vi "Access Privilege_Enable Disable Control.vi"(10 "Sidebar Ref":refnum<vi>, 11 "Previllage":string) -> ()   [LabVIEW 2023, in "GUI.lvlib"]
uses:
  GUI.lvlib
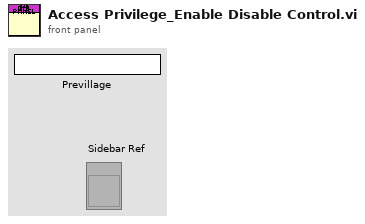
[diagram p1: front panel]
types:
  T1 = enum8{"Enabled", "Disabled", "Disabled and Grayed Out"}
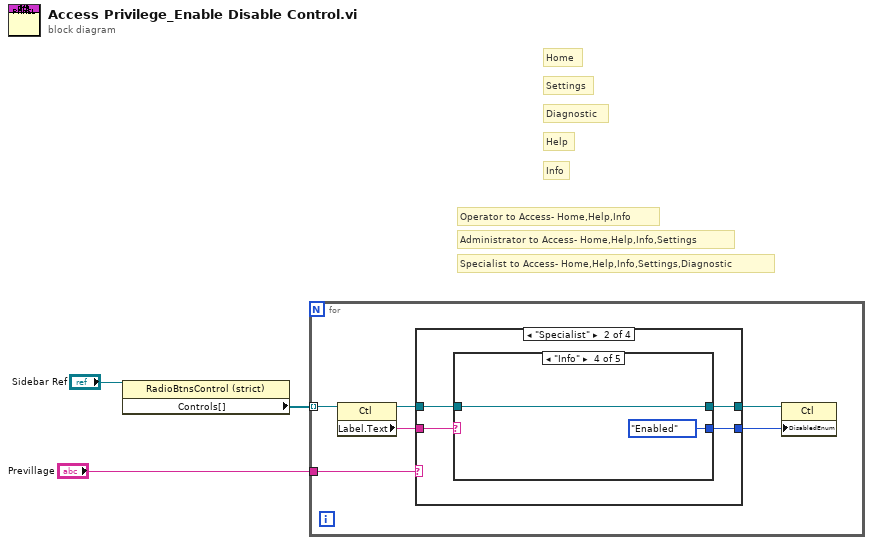
[diagram p0: block diagram]
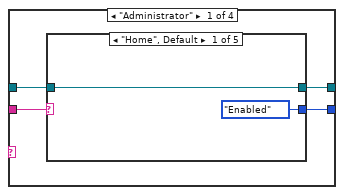
[diagram p2: hidden frame]
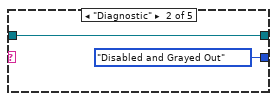
[diagram p3: hidden frame]
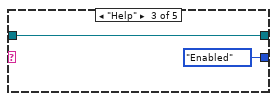
[diagram p4: hidden frame]
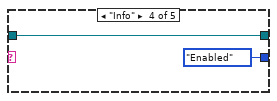
[diagram p5: hidden frame]
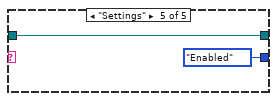
[diagram p6: hidden frame]
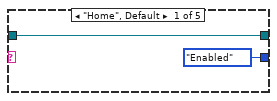
[diagram p7: hidden frame]
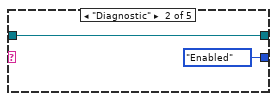
[diagram p8: hidden frame]
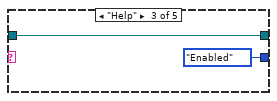
[diagram p9: hidden frame]
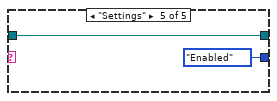
[diagram p10: hidden frame]
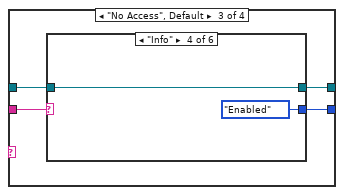
[diagram p11: hidden frame]
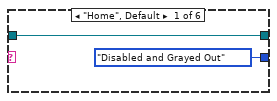
[diagram p12: hidden frame]
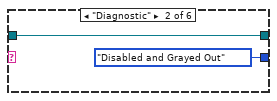
[diagram p13: hidden frame]
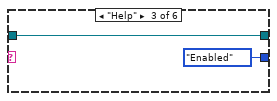
[diagram p14: hidden frame]
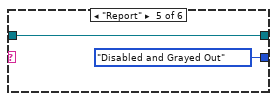
[diagram p15: hidden frame]
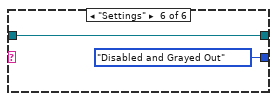
[diagram p16: hidden frame]
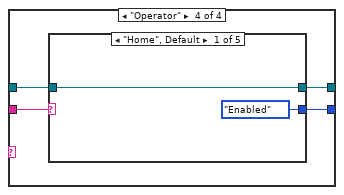
[diagram p17: hidden frame]
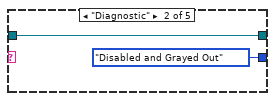
[diagram p18: hidden frame]
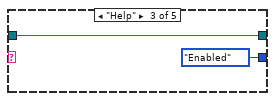
[diagram p19: hidden frame]
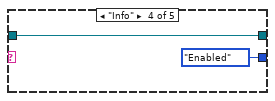
[diagram p20: hidden frame]
diagram:
  # "Specialist to Access- Home,Help,Info,Settings,Diagnostic"
  # "Administrator to Access- Home,Help,Info,Settings"
  # "Operator to Access- Home,Help,Info"
  # "Info"
  # "Help"
  # "Diagnostic"
  # "Home"
  # "Settings"
  n1 = property class="RadioBtnsControl (strict)"(reference="Sidebar Ref") -> ("Controls[]"=w3:refnum<vi>[])  [unwired: 1 in, 2 out]
  n2 = for {
    tunnel: w3 -> [w7] mode=indexing
    tunnel: "Previllage" -> [w8]
    n3 = property class="Ctl"(reference=w7) -> (reference out=w5:refnum<vi>, "Label.Text"=w6:string)  [unwired: 1 in, 1 out]
    n4 = case shown="\"Specialist\"" w8 {
      tunnel: w5 -> [w11 w25 w39 w55]
      tunnel: [w13 w27 w41 w57] -> w9
      tunnel: [w12 w26 w40 w56] -> w4
      tunnel: w6 -> [w10 w24 w38 w54]
      frame "Administrator" {
        n5 = case shown="\"Home\", Default" w10 {
          tunnel: w11 -> [w15 w17 w19 w20 w22]
          tunnel: [w15 w17 w19 w20 w22] -> w13
          tunnel: [T1."Enabled" ("Disabled") T1."Disabled and Grayed Out" ("Disabled") T1."Enabled" ("Disabled") T1."Enabled" ("Disabled") T1."Enabled" ("Disabled")] -> w12
          frame "Home", Default {
          }
          frame "Diagnostic" {
          }
          frame "Help" {
          }
          frame "Info" {
          }
          frame "Settings" {
          }
        }
      }
      frame "Specialist" {
        n6 = case shown="\"Info\"" w24 {
          tunnel: w25 -> [w29 w31 w33 w34 w36]
          tunnel: [w29 w31 w33 w34 w36] -> w27
          tunnel: [T1."Enabled" ("Disabled") T1."Enabled" ("Disabled") T1."Enabled" ("Disabled") T1."Enabled" ("Disabled") T1."Enabled" ("Disabled")] -> w26
          frame "Home", Default {
          }
          frame "Diagnostic" {
          }
          frame "Help" {
          }
          frame "Info" {
          }
          frame "Settings" {
          }
        }
      }
      frame "No Access", Default {
        n7 = case shown="\"Info\"" w38 {
          tunnel: w39 -> [w43 w45 w47 w48 w51 w52]
          tunnel: [w43 w45 w47 w48 w51 w52] -> w41
          tunnel: [T1."Disabled and Grayed Out" ("Disabled") T1."Disabled and Grayed Out" ("Disabled") T1."Enabled" ("Disabled") T1."Enabled" ("Disabled") T1."Disabled and Grayed Out" ("Disabled") T1."Disabled and Grayed Out" ("Disabled")] -> w40
          frame "Home", Default {
          }
          frame "Diagnostic" {
          }
          frame "Help" {
          }
          frame "Info" {
          }
          frame "Report" {
          }
          frame "Settings" {
          }
        }
      }
      frame "Operator" {
        n8 = case shown="\"Home\", Default" w54 {
          tunnel: w55 -> [w59 w61 w63 w64 w66]
          tunnel: [w59 w61 w63 w64 w66] -> w57
          tunnel: [T1."Enabled" ("Disabled") T1."Disabled and Grayed Out" ("Disabled") T1."Enabled" ("Disabled") T1."Enabled" ("Disabled") T1."Disabled and Grayed Out" ("Disabled")] -> w56
          frame "Home", Default {
          }
          frame "Diagnostic" {
          }
          frame "Help" {
          }
          frame "Info" {
          }
          frame "Settings" {
          }
        }
      }
    }
    n9 = property class="Ctl"(reference=w9, "DisabledEnum"=w4) -> ()  [unwired: 1 in, 2 out]
  }
